vi "Autonomous Independent.vi"() -> ()   [LabVIEW 2015]
doc: "This VI is called when autonomous begins, and will automatically be terminated when autonomous ends. You can carry out timed or sensor driven robot movement independently without needing to return to the caller."
uses:
  Autonomous movements.ctl
  Mode for autonomous.ctl
  <vilib>/Rock Robotics/WPI/Utilities/WPI_GetSetVariantRefNum.vi
  <vilib>/Rock Robotics/Network Tables/NT Read String.vi
  <vilib>/Rock Robotics/Network Tables/NT Write Numeric Array.vi
  <vilib>/Rock Robotics/Network Tables/SD Write String.vi
  <vilib>/Rock Robotics/WPI/RobotDrive/WPI_RobotDriveArcadeDrive_Standard(NoSaturation).vi
  <vilib>/Rock Robotics/Network Tables/SD Write Numeric Array.vi
panel:
  in  "shoot low goal O5 (any)":T1[](array[typedef])=[{"X Joystick Value"=0.0, "Y Joystick Value"=-0.3673469387755101, "Z Joystick Value"=0.0, "Delay (sec)"=4.0, "Movement Name"="", "Mode"=enum."Move Robot"}, {"X Joystick Value"=-0.313131, "Y Joystick Value"=0.0, "Z Joystick Value"=0.0, "Delay (sec)"=1.5, "Movement Name"="", "Mode"=enum."Move Robot"}, {"X Joystick Value"=0.0, "Y Joystick Value"=-0.3, "Z Joystick Value"=0.0, "Delay (sec)"=3.5, "Movement Name"="", "Mode"=enum."Move Robot"}, {"X Joystick Value"=0.373737, "Y Joystick Value"=0.0, "Z Joystick Value"=0.0, "Delay (sec)"=1.5, "Movement Name"="", "Mode"=enum."Move Robot"}, {"X Joystick Value"=0.0, "Y Joystick Value"=-0.3673469387755101, "Z Joystick Value"=0.0, "Delay (sec)"=1.5, "Movement Name"="", "Mode"=enum."Move Robot"}, {"X Joystick Value"=0.0, "Y Joystick Value"=0.0, "Z Joystick Value"=0.0, "Delay (sec)"=2.5, "Movement Name"="", "Mode"=enum."Shoot Low Goal"}, {"X Joystick Value"=0.0, "Y Joystick Value"=-1.0, "Z Joystick Value"=0.0, "Delay (sec)"=0.0, "Movement Name"="", "Mode"=enum."Move Robot"}, {"X Joystick Value"=-1.0, "Y Joystick Value"=0.0, "Z Joystick Value"=0.0, "Delay (sec)"=0.0, "Movement Name"="", "Mode"=enum."Do Nothing"}, {"X Joystick Value"=0.0, "Y Joystick Value"=-1.0, "Z Joystick Value"=0.0, "Delay (sec)"=0.0, "Movement Name"="", "Mode"=enum."Do Nothing"}, {"X Joystick Value"=0.0, "Y Joystick Value"=0.0, "Z Joystick Value"=0.0, "Delay (sec)"=5.0, "Movement Name"="", "Mode"=enum."Do Nothing"}, {"X Joystick Value"=0.0, "Y Joystick Value"=-1.0, "Z Joystick Value"=0.0, "Delay (sec)"=0.0, "Movement Name"="", "Mode"=enum."Do Nothing"}, {"X Joystick Value"=0.0, "Y Joystick Value"=0.0, "Z Joystick Value"=0.0, "Delay (sec)"=0.0, "Movement Name"="", "Mode"=enum."Do Nothing"}] {"Z Joystick Value" scale=-1.0..1.0; "Y Joystick Value" scale=1.0..-1.0; "X Joystick Value" scale=-1.0..1.0}
  in  "shoot low goal O4 (any)":T1[](array[typedef])=[{"X Joystick Value"=0.0, "Y Joystick Value"=-0.3673469387755101, "Z Joystick Value"=0.0, "Delay (sec)"=4.0, "Movement Name"="", "Mode"=enum."Move Robot"}, {"X Joystick Value"=-0.313131, "Y Joystick Value"=0.0, "Z Joystick Value"=0.0, "Delay (sec)"=1.5, "Movement Name"="", "Mode"=enum."Move Robot"}, {"X Joystick Value"=0.0, "Y Joystick Value"=-0.3, "Z Joystick Value"=0.0, "Delay (sec)"=3.5, "Movement Name"="", "Mode"=enum."Move Robot"}, {"X Joystick Value"=0.373737, "Y Joystick Value"=0.0, "Z Joystick Value"=0.0, "Delay (sec)"=0.75, "Movement Name"="", "Mode"=enum."Move Robot"}, {"X Joystick Value"=0.0, "Y Joystick Value"=-0.3673469387755101, "Z Joystick Value"=0.0, "Delay (sec)"=1.5, "Movement Name"="", "Mode"=enum."Move Robot"}, {"X Joystick Value"=0.0, "Y Joystick Value"=0.0, "Z Joystick Value"=0.0, "Delay (sec)"=2.5, "Movement Name"="", "Mode"=enum."Shoot Low Goal"}, {"X Joystick Value"=0.0, "Y Joystick Value"=-1.0, "Z Joystick Value"=0.0, "Delay (sec)"=0.0, "Movement Name"="", "Mode"=enum."Move Robot"}, {"X Joystick Value"=-1.0, "Y Joystick Value"=0.0, "Z Joystick Value"=0.0, "Delay (sec)"=0.0, "Movement Name"="", "Mode"=enum."Do Nothing"}, {"X Joystick Value"=0.0, "Y Joystick Value"=-1.0, "Z Joystick Value"=0.0, "Delay (sec)"=0.0, "Movement Name"="", "Mode"=enum."Do Nothing"}, {"X Joystick Value"=0.0, "Y Joystick Value"=0.0, "Z Joystick Value"=0.0, "Delay (sec)"=5.0, "Movement Name"="", "Mode"=enum."Do Nothing"}, {"X Joystick Value"=0.0, "Y Joystick Value"=-1.0, "Z Joystick Value"=0.0, "Delay (sec)"=0.0, "Movement Name"="", "Mode"=enum."Do Nothing"}, {"X Joystick Value"=0.0, "Y Joystick Value"=0.0, "Z Joystick Value"=0.0, "Delay (sec)"=0.0, "Movement Name"="", "Mode"=enum."Do Nothing"}] {"Z Joystick Value" scale=-1.0..1.0; "Y Joystick Value" scale=1.0..-1.0; "X Joystick Value" scale=-1.0..1.0}
  in  "shoot low goal O3 (any)":T1[](array[typedef])=[{"X Joystick Value"=0.0, "Y Joystick Value"=-0.3673469387755101, "Z Joystick Value"=0.0, "Delay (sec)"=4.0, "Movement Name"="", "Mode"=enum."Move Robot"}, {"X Joystick Value"=0.31313131313131326, "Y Joystick Value"=0.0, "Z Joystick Value"=0.0, "Delay (sec)"=1.5, "Movement Name"="", "Mode"=enum."Move Robot"}, {"X Joystick Value"=0.0, "Y Joystick Value"=-0.3, "Z Joystick Value"=0.0, "Delay (sec)"=3.5, "Movement Name"="", "Mode"=enum."Move Robot"}, {"X Joystick Value"=-0.373737, "Y Joystick Value"=0.0, "Z Joystick Value"=0.0, "Delay (sec)"=0.75, "Movement Name"="", "Mode"=enum."Move Robot"}, {"X Joystick Value"=0.0, "Y Joystick Value"=-0.3673469387755101, "Z Joystick Value"=0.0, "Delay (sec)"=1.5, "Movement Name"="", "Mode"=enum."Move Robot"}, {"X Joystick Value"=0.0, "Y Joystick Value"=0.0, "Z Joystick Value"=0.0, "Delay (sec)"=2.5, "Movement Name"="", "Mode"=enum."Shoot Low Goal"}, {"X Joystick Value"=0.0, "Y Joystick Value"=-1.0, "Z Joystick Value"=0.0, "Delay (sec)"=0.0, "Movement Name"="", "Mode"=enum."Move Robot"}, {"X Joystick Value"=-1.0, "Y Joystick Value"=0.0, "Z Joystick Value"=0.0, "Delay (sec)"=0.0, "Movement Name"="", "Mode"=enum."Do Nothing"}, {"X Joystick Value"=0.0, "Y Joystick Value"=-1.0, "Z Joystick Value"=0.0, "Delay (sec)"=0.0, "Movement Name"="", "Mode"=enum."Do Nothing"}, {"X Joystick Value"=0.0, "Y Joystick Value"=0.0, "Z Joystick Value"=0.0, "Delay (sec)"=5.0, "Movement Name"="", "Mode"=enum."Do Nothing"}, {"X Joystick Value"=0.0, "Y Joystick Value"=-1.0, "Z Joystick Value"=0.0, "Delay (sec)"=0.0, "Movement Name"="", "Mode"=enum."Do Nothing"}, {"X Joystick Value"=0.0, "Y Joystick Value"=0.0, "Z Joystick Value"=0.0, "Delay (sec)"=0.0, "Movement Name"="", "Mode"=enum."Do Nothing"}] {"Z Joystick Value" scale=-1.0..1.0; "Y Joystick Value" scale=1.0..-1.0; "X Joystick Value" scale=-1.0..1.0}
  in  "shoot low goal O2 (any)":T1[](array[typedef])=[{"X Joystick Value"=0.0, "Y Joystick Value"=-0.3673469387755101, "Z Joystick Value"=0.0, "Delay (sec)"=4.0, "Movement Name"="", "Mode"=enum."Move Robot"}, {"X Joystick Value"=0.31313131313131326, "Y Joystick Value"=0.0, "Z Joystick Value"=0.0, "Delay (sec)"=1.5, "Movement Name"="", "Mode"=enum."Move Robot"}, {"X Joystick Value"=0.0, "Y Joystick Value"=-0.3, "Z Joystick Value"=0.0, "Delay (sec)"=3.5, "Movement Name"="", "Mode"=enum."Move Robot"}, {"X Joystick Value"=-0.373737, "Y Joystick Value"=0.0, "Z Joystick Value"=0.0, "Delay (sec)"=1.5, "Movement Name"="", "Mode"=enum."Move Robot"}, {"X Joystick Value"=0.0, "Y Joystick Value"=-0.3673469387755101, "Z Joystick Value"=0.0, "Delay (sec)"=1.5, "Movement Name"="", "Mode"=enum."Move Robot"}, {"X Joystick Value"=0.0, "Y Joystick Value"=0.0, "Z Joystick Value"=0.0, "Delay (sec)"=2.5, "Movement Name"="", "Mode"=enum."Shoot Low Goal"}, {"X Joystick Value"=0.0, "Y Joystick Value"=-1.0, "Z Joystick Value"=0.0, "Delay (sec)"=0.0, "Movement Name"="", "Mode"=enum."Move Robot"}, {"X Joystick Value"=-1.0, "Y Joystick Value"=0.0, "Z Joystick Value"=0.0, "Delay (sec)"=0.0, "Movement Name"="", "Mode"=enum."Do Nothing"}, {"X Joystick Value"=0.0, "Y Joystick Value"=-1.0, "Z Joystick Value"=0.0, "Delay (sec)"=0.0, "Movement Name"="", "Mode"=enum."Do Nothing"}, {"X Joystick Value"=0.0, "Y Joystick Value"=0.0, "Z Joystick Value"=0.0, "Delay (sec)"=5.0, "Movement Name"="", "Mode"=enum."Do Nothing"}, {"X Joystick Value"=0.0, "Y Joystick Value"=-1.0, "Z Joystick Value"=0.0, "Delay (sec)"=0.0, "Movement Name"="", "Mode"=enum."Do Nothing"}, {"X Joystick Value"=0.0, "Y Joystick Value"=0.0, "Z Joystick Value"=0.0, "Delay (sec)"=0.0, "Movement Name"="", "Mode"=enum."Do Nothing"}] {"Z Joystick Value" scale=-1.0..1.0; "Y Joystick Value" scale=1.0..-1.0; "X Joystick Value" scale=-1.0..1.0}
  in  "shoot low goal O1.":T1[](array[typedef])=[{"X Joystick Value"=0.0, "Y Joystick Value"=-0.3673469387755101, "Z Joystick Value"=0.0, "Delay (sec)"=4.0, "Movement Name"="", "Mode"=enum."Move Robot"}, {"X Joystick Value"=0.31313131313131326, "Y Joystick Value"=0.0, "Z Joystick Value"=0.0, "Delay (sec)"=1.5, "Movement Name"="", "Mode"=enum."Move Robot"}, {"X Joystick Value"=0.0, "Y Joystick Value"=-0.3, "Z Joystick Value"=0.0, "Delay (sec)"=4.0, "Movement Name"="", "Mode"=enum."Move Robot"}, {"X Joystick Value"=-0.373737, "Y Joystick Value"=0.0, "Z Joystick Value"=0.0, "Delay (sec)"=1.5, "Movement Name"="", "Mode"=enum."Move Robot"}, {"X Joystick Value"=0.0, "Y Joystick Value"=-0.3673469387755101, "Z Joystick Value"=0.0, "Delay (sec)"=1.5, "Movement Name"="", "Mode"=enum."Move Robot"}, {"X Joystick Value"=0.0, "Y Joystick Value"=0.0, "Z Joystick Value"=0.0, "Delay (sec)"=2.5, "Movement Name"="", "Mode"=enum."Shoot Low Goal"}, {"X Joystick Value"=0.0, "Y Joystick Value"=-1.0, "Z Joystick Value"=0.0, "Delay (sec)"=0.0, "Movement Name"="", "Mode"=enum."Move Robot"}, {"X Joystick Value"=-1.0, "Y Joystick Value"=0.0, "Z Joystick Value"=0.0, "Delay (sec)"=0.0, "Movement Name"="", "Mode"=enum."Do Nothing"}, {"X Joystick Value"=0.0, "Y Joystick Value"=-1.0, "Z Joystick Value"=0.0, "Delay (sec)"=0.0, "Movement Name"="", "Mode"=enum."Do Nothing"}, {"X Joystick Value"=0.0, "Y Joystick Value"=0.0, "Z Joystick Value"=0.0, "Delay (sec)"=5.0, "Movement Name"="", "Mode"=enum."Do Nothing"}, {"X Joystick Value"=0.0, "Y Joystick Value"=-1.0, "Z Joystick Value"=0.0, "Delay (sec)"=0.0, "Movement Name"="", "Mode"=enum."Do Nothing"}, {"X Joystick Value"=0.0, "Y Joystick Value"=0.0, "Z Joystick Value"=0.0, "Delay (sec)"=0.0, "Movement Name"="", "Mode"=enum."Do Nothing"}] {"Z Joystick Value" scale=-1.0..1.0; "Y Joystick Value" scale=1.0..-1.0; "X Joystick Value" scale=-1.0..1.0}
  in  "move forward":T1[](array[typedef])=[{"X Joystick Value"=0.0, "Y Joystick Value"=-0.3, "Z Joystick Value"=0.0, "Delay (sec)"=2.5, "Movement Name"="", "Mode"=enum."Move Robot"}, {"X Joystick Value"=0.0, "Y Joystick Value"=0.0, "Z Joystick Value"=0.0, "Delay (sec)"=5.0, "Movement Name"="", "Mode"=enum."Move Robot"}, {"X Joystick Value"=0.0, "Y Joystick Value"=-1.0, "Z Joystick Value"=0.0, "Delay (sec)"=0.0, "Movement Name"="", "Mode"=enum."Move Robot"}, {"X Joystick Value"=-1.0, "Y Joystick Value"=0.0, "Z Joystick Value"=0.0, "Delay (sec)"=5.0, "Movement Name"="", "Mode"=enum."Do Nothing"}, {"X Joystick Value"=0.0, "Y Joystick Value"=-1.0, "Z Joystick Value"=0.0, "Delay (sec)"=0.0, "Movement Name"="", "Mode"=enum."Do Nothing"}, {"X Joystick Value"=0.0, "Y Joystick Value"=0.0, "Z Joystick Value"=0.0, "Delay (sec)"=0.0, "Movement Name"="", "Mode"=enum."Do Nothing"}, {"X Joystick Value"=0.0, "Y Joystick Value"=-1.0, "Z Joystick Value"=0.0, "Delay (sec)"=0.0, "Movement Name"="", "Mode"=enum."Move Robot"}, {"X Joystick Value"=-1.0, "Y Joystick Value"=0.0, "Z Joystick Value"=0.0, "Delay (sec)"=0.0, "Movement Name"="", "Mode"=enum."Do Nothing"}, {"X Joystick Value"=0.0, "Y Joystick Value"=-1.0, "Z Joystick Value"=0.0, "Delay (sec)"=0.0, "Movement Name"="", "Mode"=enum."Do Nothing"}, {"X Joystick Value"=0.0, "Y Joystick Value"=0.0, "Z Joystick Value"=0.0, "Delay (sec)"=5.0, "Movement Name"="", "Mode"=enum."Do Nothing"}, {"X Joystick Value"=0.0, "Y Joystick Value"=-1.0, "Z Joystick Value"=0.0, "Delay (sec)"=0.0, "Movement Name"="", "Mode"=enum."Do Nothing"}, {"X Joystick Value"=0.0, "Y Joystick Value"=0.0, "Z Joystick Value"=0.0, "Delay (sec)"=0.0, "Movement Name"="", "Mode"=enum."Do Nothing"}] {"Z Joystick Value" scale=-1.0..1.0; "Y Joystick Value" scale=1.0..-1.0; "X Joystick Value" scale=-1.0..1.0}
  in  "do nothing":T1[](array[typedef])=[{"X Joystick Value"=0.0, "Y Joystick Value"=0.0, "Z Joystick Value"=0.0, "Delay (sec)"=15.0, "Movement Name"="", "Mode"=enum."Do Nothing"}] {"Z Joystick Value" scale=-1.0..1.0; "Y Joystick Value" scale=1.0..-1.0; "X Joystick Value" scale=-1.0..1.0}
  out "Current Movement, for debugging":T3 {"Y Joystick Value" scale=1.0..-1.0; "X Joystick Value" scale=-1.0..1.0}
  in  "Array of robot movements":T4(array[cluster])=[{"X Joystick Value"=0.39393939393939403, "Y Joystick Value"=0.0, "Delay (sec)"=1.0, "Movement Name"="turn"}, {"X Joystick Value"=-0.3737373737373737, "Y Joystick Value"=0.0, "Delay (sec)"=1.0, "Movement Name"="turn back"}] {"Y Joystick Value" scale=1.0..-1.0; "X Joystick Value" scale=-1.0..1.0}
  # "Be sure to right-click and choose Data Operations>>Make Current Value default if you want to save the array values with the VI"
  # "start in position one"
  # "DONT USE Z VALUE\n\nSET CURRENT VALUES AS DEFAULT"
  # "move forward"
  # "shoot low goal"
  # "move forward"
  # "turn left"
  # "turn right"
  # "move forward"
  # "move forward"
  # "turn right"
  # "move forward"
  # "turn left"
  # "shoot low goal"
  # "move forward"
  # "move forward"
  # "turn right"
  # "move forward"
  # "turn left"
  # "shoot low goal"
  # "move forward"
  # "move forward"
  # "turn left"
  # "move forward"
  # "turn right"
  # "shoot low goal"
  # "move forward"
  # "move forward"
  # "move forward"
  # "turn left"
  # "move forward"
  # "turn right"
  # "shoot low goal"
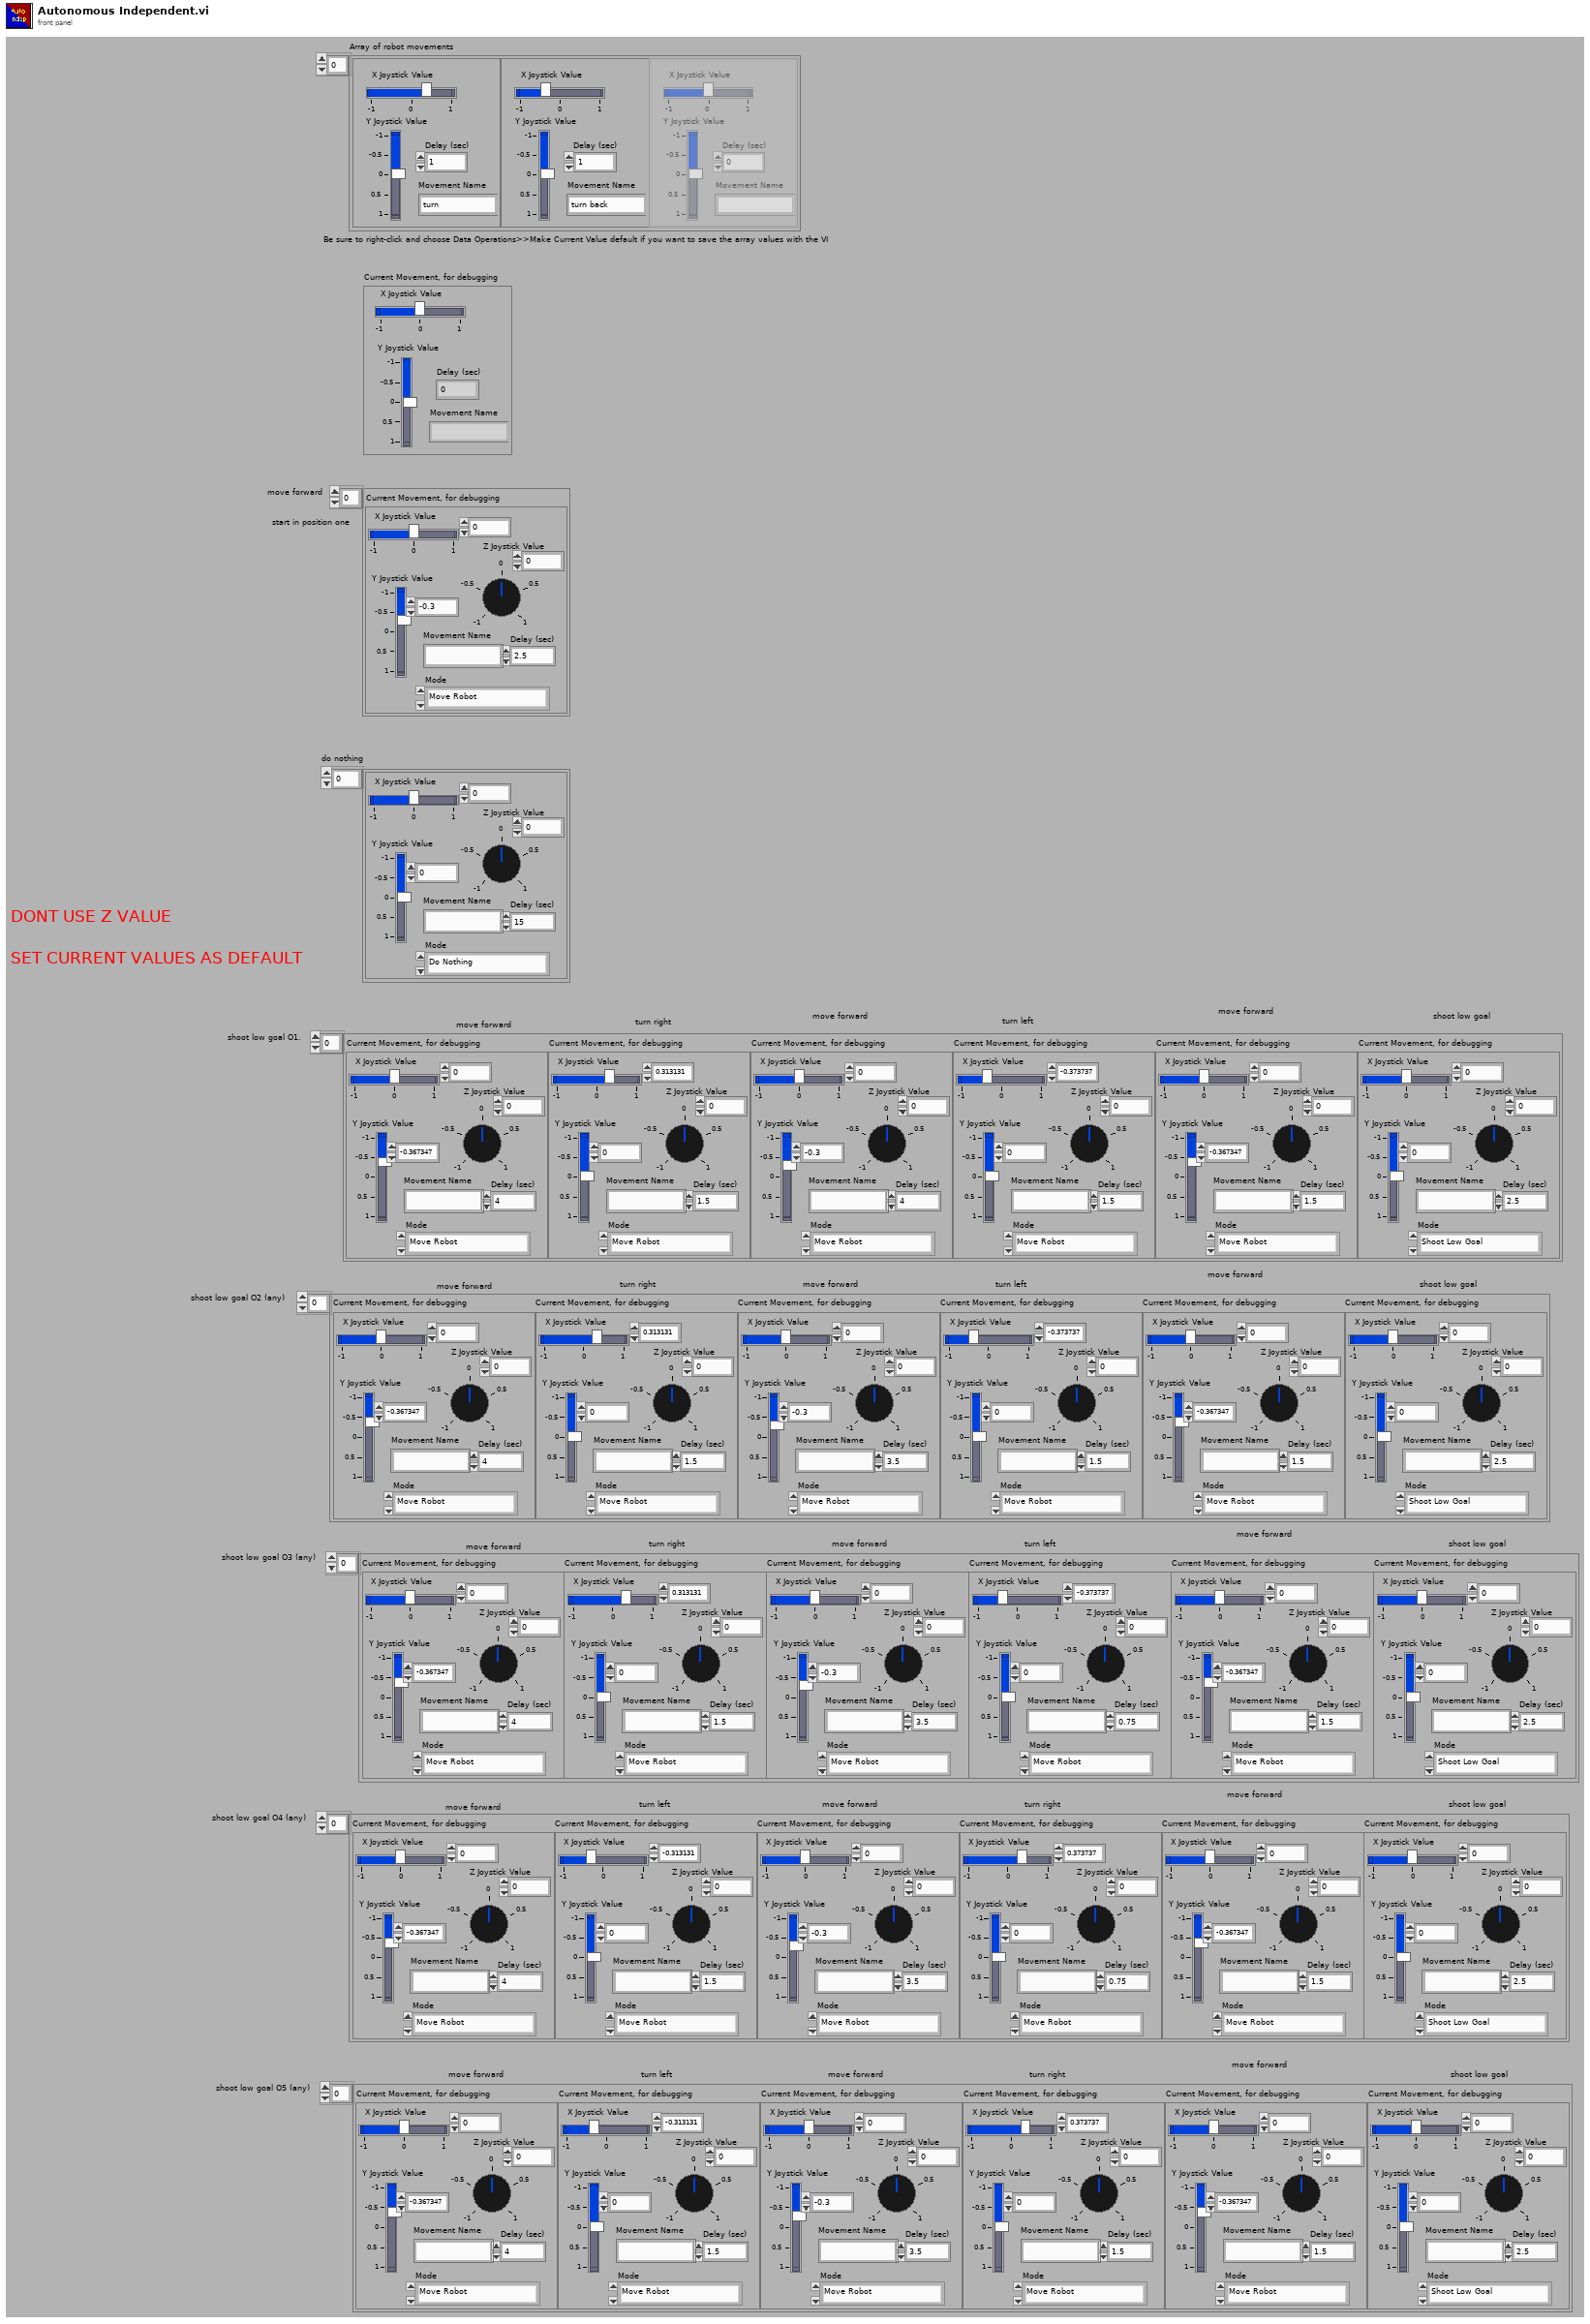
[diagram p1: front panel]
types:
  T1 = typedef "Autonomous movements.ctl" = cluster{"X Joystick Value":dbl, "Y Joystick Value":dbl, "Z Joystick Value":dbl, "Delay (sec)":dbl, "Movement Name":string, "Mode":T2}
  T2 = typedef "Mode for autonomous.ctl" = enum16{"Do Nothing", "Move Robot", "Shoot Low Goal", "Shoot High Goal"}
  T3 = cluster{"X Joystick Value":dbl, "Y Joystick Value":dbl, "Delay (sec)":dbl, "Movement Name":string}
  T4 = cluster{"X Joystick Value":dbl, "Y Joystick Value":dbl, "Delay (sec)":dbl, "Movement Name":string}[]
  T5 = typedef "WPI_JoystickDevRef.ctl" = cluster{"Device":T6}
  T6 = typedef "WPI_JoystickDeviceEnum.ctl" = enum16{"USB 0", "USB 1", "USB 2", "USB 3", "USB 4", "USB 5"}
  T7 = typedef "WPI_RobotDriveDevRef.ctl" = cluster{"DevStatus":errorcluster, "Motors[]":T8[], "Square Inputs":bool, "Max Output":dbl}
  T8 = typedef "WPI_MotorControlDeviceRef.ctl" = cluster{"DeviceStatus":errorcluster, "Type":T9, "PWM":cluster{"PWM Channel":T10, "DeadBand":T11}, "CAN":cluster{"Device Number":u8, "Control Mode":T12, "Semaphore":T13, "Max Vout":dbl, "TalonSRX Control Mode":T14}, "Invert":bool}
  T9 = typedef "WPI_MotorControlType.ctl" = enum16{"PWM", "CAN", "CANTalonSRX"}
  T10 = typedef "FPGA_DIOPWMChannel.ctl" = enum8{"PWM 0", "PWM 1", "PWM 2", "PWM 3", "PWM 4", "PWM 5", "PWM 6", "PWM 7", "PWM 8", "PWM 9", "PWM MXP 0", "PWM MXP 1", "PWM MXP 2", "PWM MXP 3", "PWM MXP 4", "PWM MXP 5", "PWM MXP 6", "PWM MXP 7", "PWM MXP 8", "PWM MXP 9", "Invalid"}
  T11 = typedef "WPI_PWMDeadband.ctl" = cluster{"Name":string, "maxPositivePwm":i32, "minPositivePwm":i32, "centerPwm":i32, "maxNegativePwm":i32, "minNegativePwm":i32, "angularRange":u16}
  T12 = typedef "WPI_CANJaguar_ControlMode.ctl" = enum8{"Percent VBus", "Current", "Speed", "Position", "Voltage"}
  T13 = typedef "Semaphore RefNum" = refnum<k1>
  T14 = typedef "WPI_CANTalonSRX_APIControlMode.ctl" = enum8{"Percent VBus", "Speed", "Position", "Slave", "Unchanged / Invalid", "Voltage Compensation", "Current", "Motion Profile"}
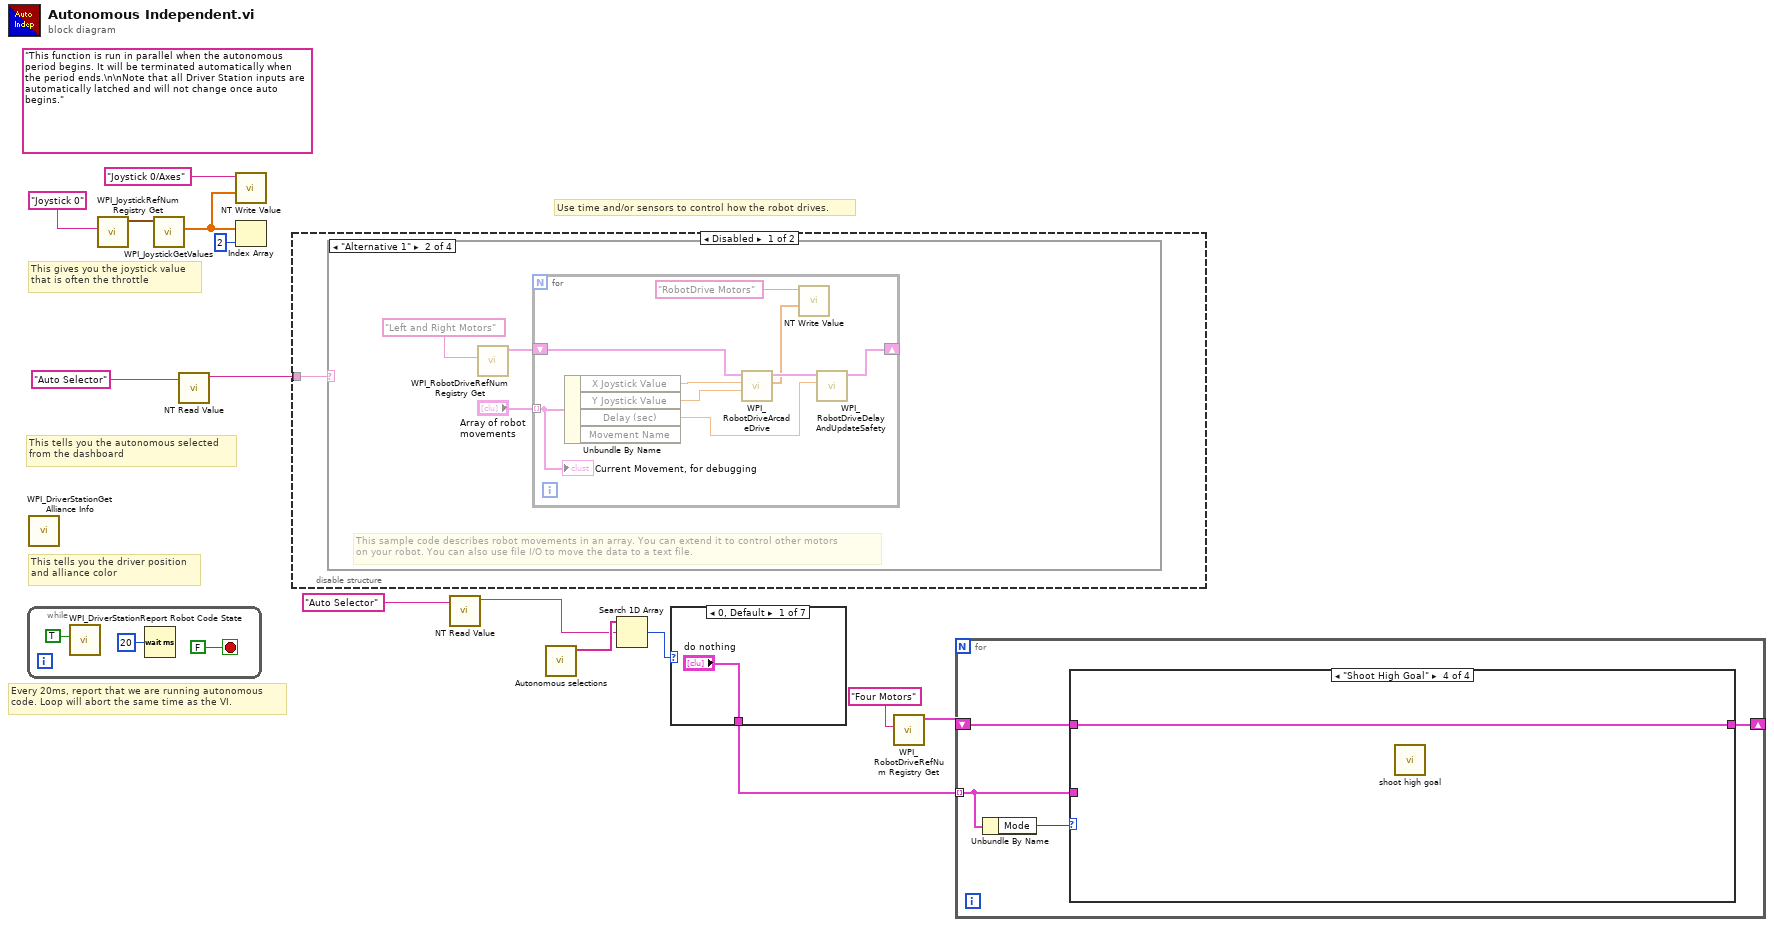
[diagram p0: block diagram]
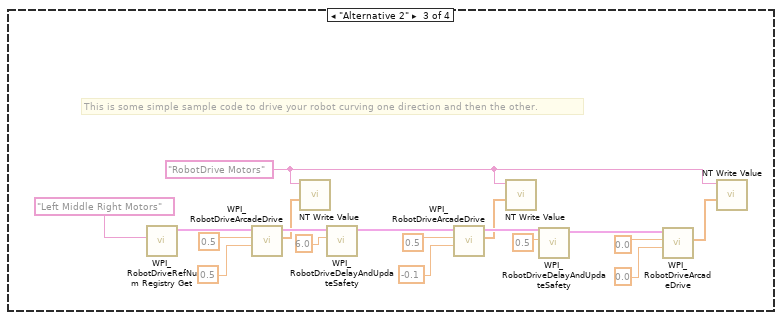
[diagram p3: hidden frame]
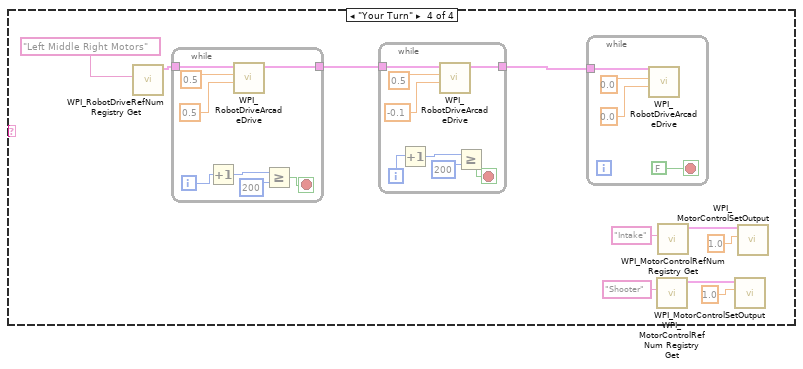
[diagram p4: hidden frame]
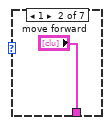
[diagram p6: hidden frame]
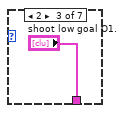
[diagram p7: hidden frame]
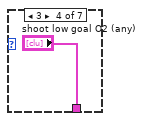
[diagram p8: hidden frame]
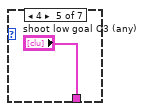
[diagram p9: hidden frame]
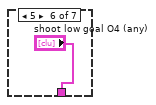
[diagram p10: hidden frame]
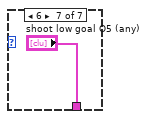
[diagram p11: hidden frame]
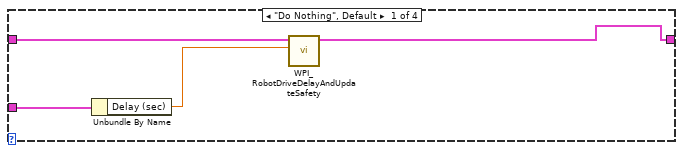
[diagram p12: hidden frame]
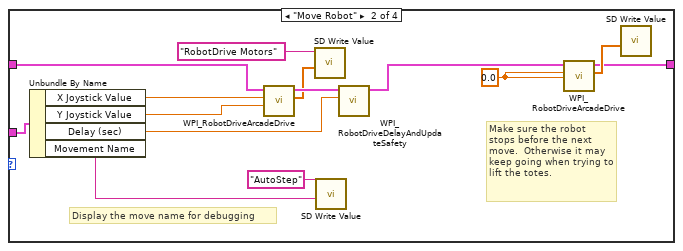
[diagram p13: hidden frame]
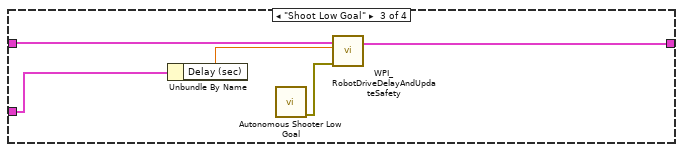
[diagram p14: hidden frame]
diagram:
  (unwired) "This function is run in parallel when the autonomous period begins. It will be terminated automatically when the period ends.\n\nNote that all Driver Station inputs are automatically latched and will not change once auto begins."
  # "This tells you the autonomous selected\nfrom the dashboard"
  # "Every 20ms, report that we are running autonomous\ncode. Loop will abort the same time as the VI."
  # "This gives you the joystick value\nthat is often the throttle"
  # "Use time and/or sensors to control how the robot drives."
  # "This tells you the driver position\nand alliance color"
  n1 = while {
    stop <- FALSE stop-if-true
    n2 = call <vilib>:"WPI_DriverStationReport Robot Code State.vi"("Autonomous"=TRUE) -> ()  [unwired: 10 in, 1 out]
    n3 = Wait (ms)(milliseconds to wait=u32 20) -> ()  [unwired: 1 out]
  }
  n4 = call <vilib>:"WPI_DriverStationGet Alliance Info.vi"() -> ()  [unwired: 12 out]
  n5 = call <vilib>:"WPI_JoystickRefNum Registry Get.vi"("refnum name"="Joystick 0") -> ("JoystickDevRef"=w13:T5)  [unwired: 1 in, 9 out]
  n6 = call <vilib>:"WPI_JoystickGetValues.vi"("JoystickDevRef"=w13) -> ("Axes"=w9:dbl[])  [unwired: 6 in, 4 out]
  n7 = call-poly <vilib>:"NT Read Value.vi"("Name"="Auto Selector") -> ("String"=w10:string)  [unwired: 9 in, 1 out]
  n8 = call-poly <vilib>:"NT Write Value.vi"("Numeric Array"=w9, "Name"="Joystick 0/Axes") -> ()  [unwired: 9 in, 1 out]
  n9 = Index Array(array=w9, index=2) -> ()  [unwired: 1 out]
  n10 = disable-structure shown="Disabled" {
    disable-tunnel: w10 -> [w18 _]
    frame Disabled {
      n11 = case shown="\"Alternative 1\"" w18 {
        frame Default {
          # "You can put your main auto here, or you can right-click on the case and make any\nother frame be the default case."
          # "This is the frame that will execute if no selection is made, or if it is not recognized"
        }
        frame "Alternative 1" {
          # "This sample code describes robot movements in an array. You can extend it to control other motors\non your robot. You can also use file I/O to move the data to a text file."
          n12 = call <vilib>:"WPI_RobotDriveRefNum Registry Get.vi"("refnum name"="Left and Right Motors") -> ("RobotDriveDevRef"=w20:T7)  [unwired: 1 in, 9 out]
          n13 = for {
            shift-right: [w28] -> _
            shift-left: w20 -> [w29]
            tunnel: "Array of robot movements" -> [w24] mode=indexing
            n14 = Unbundle By Name(w24) -> ("X Joystick Value"=w27:dbl, "Y Joystick Value"=w26:dbl, "Delay (sec)"=w25:dbl)  [unwired: 1 out]
            n15 = call-poly <vilib>:"WPI_RobotDriveArcadeDrive.vi"("Y axis value"=w26, "X axis value"=w27, "RobotDriveDevRef"=w29) -> ("Motor Values"=w22:dbl[], "RobotDriveDevRef"=w30:T7)  [unwired: 1 in, 6 out]
            n16 = call-poly <vilib>:"NT Write Value.vi"("Numeric Array"=w22, "Name"="RobotDrive Motors") -> ()  [unwired: 9 in, 1 out]
            n17 = call <vilib>:"WPI_RobotDriveDelayAndUpdateSafety.vi"("Delay (s)"=w25, "RobotDriveDevRef"=w30) -> ("RobotDriveDevRef 2"=w28:T7)  [unwired: 8 in, 1 out]
            "Current Movement, for debugging" <- w24
          }
        }
        frame "Alternative 2" {
          w32 = "RobotDrive Motors" ("Name")
          # "This is some simple sample code to drive your robot curving one direction and then the other."
          n18 = call <vilib>:"WPI_RobotDriveRefNum Registry Get.vi"("refnum name"="Left Middle Right Motors") -> ("RobotDriveDevRef"=w48:T7)  [unwired: 1 in, 9 out]
          n19 = call-poly <vilib>:"WPI_RobotDriveArcadeDrive.vi"("Y axis value"=0.5 ("X axis value"), "X axis value"=0.5, "RobotDriveDevRef"=w48) -> ("Motor Values"=w31:dbl[], "RobotDriveDevRef"=w41:T7)  [unwired: 1 in, 6 out]
          n20 = call-poly <vilib>:"NT Write Value.vi"("Numeric Array"=w31, "Name"=w32) -> ()  [unwired: 9 in, 1 out]
          n21 = call <vilib>:"WPI_RobotDriveDelayAndUpdateSafety.vi"("Delay (s)"=6.0, "RobotDriveDevRef"=w41) -> ("RobotDriveDevRef 2"=w42:T7)  [unwired: 8 in, 1 out]
          n22 = call-poly <vilib>:"WPI_RobotDriveArcadeDrive.vi"("Y axis value"=-0.1 ("X axis value"), "X axis value"=0.5, "RobotDriveDevRef"=w42) -> ("Motor Values"=w33:dbl[], "RobotDriveDevRef"=w43:T7)  [unwired: 1 in, 6 out]
          n23 = call-poly <vilib>:"NT Write Value.vi"("Numeric Array"=w33, "Name"=w32) -> ()  [unwired: 9 in, 1 out]
          n24 = call <vilib>:"WPI_RobotDriveDelayAndUpdateSafety.vi"("Delay (s)"=0.5, "RobotDriveDevRef"=w43) -> ("RobotDriveDevRef 2"=w44:T7)  [unwired: 8 in, 1 out]
          n25 = call-poly <vilib>:"WPI_RobotDriveArcadeDrive.vi"("Y axis value"=0.0 ("X axis value"), "X axis value"=0.0, "RobotDriveDevRef"=w44) -> ("Motor Values"=w34:dbl[])  [unwired: 1 in, 7 out]
          n26 = call-poly <vilib>:"NT Write Value.vi"("Numeric Array"=w34, "Name"=w32) -> ()  [unwired: 9 in, 1 out]
        }
        frame "Your Turn" {
          n27 = call <vilib>:"WPI_RobotDriveRefNum Registry Get.vi"("refnum name"="Left Middle Right Motors") -> ("RobotDriveDevRef"=w58:T7)  [unwired: 1 in, 9 out]
          n28 = while {
            tunnel: w58 -> [w78]
            tunnel: [w75] -> w50
            i -> [w74]
            stop <- w71 stop-if-true
            n29 = Increment(x=w74) -> (x+1=w73:i32)
            n30 = call-poly <vilib>:"WPI_RobotDriveArcadeDrive.vi"("Y axis value"=0.5 ("X axis value"), "X axis value"=0.5, "RobotDriveDevRef"=w78) -> ("RobotDriveDevRef"=w75:T7)  [unwired: 1 in, 7 out]
            n31 = Greater Or Equal?(x=w73, y=200) -> (x >= y?=w71:bool)
          }
          n32 = while {
            tunnel: w50 -> [w68]
            tunnel: [w67] -> w49
            i -> [w64]
            stop <- w63 stop-if-true
            n33 = Increment(x=w64) -> (x+1=w66:i32)
            n34 = call-poly <vilib>:"WPI_RobotDriveArcadeDrive.vi"("Y axis value"=-0.1 ("X axis value"), "X axis value"=0.5, "RobotDriveDevRef"=w68) -> ("RobotDriveDevRef"=w67:T7)  [unwired: 1 in, 7 out]
            n35 = Greater Or Equal?(x=w66, y=200) -> (x >= y?=w63:bool)
          }
          n36 = while {
            tunnel: w49 -> [w60]
            stop <- FALSE stop-if-true
            n37 = call-poly <vilib>:"WPI_RobotDriveArcadeDrive.vi"("Y axis value"=0.0 ("X axis value"), "X axis value"=0.0, "RobotDriveDevRef"=w60) -> ()  [unwired: 1 in, 8 out]
          }
          n38 = call <vilib>:"WPI_MotorControlRefNum Registry Get.vi"("refnum name"="Shooter") -> ("MotorControlDevRef"=w55:T8)  [unwired: 9 in, 1 out]
          n39 = call <vilib>:"WPI_MotorControlRefNum Registry Get.vi"("refnum name"="Intake") -> ("MotorControlDevRef"=w52:T8)  [unwired: 9 in, 1 out]
          n40 = call <vilib>:"WPI_MotorControlSetOutput.vi"("Output"=1.0, "MotorControlDevRef"=w55) -> ()  [unwired: 7 in, 3 out]
          n41 = call <vilib>:"WPI_MotorControlSetOutput.vi"("Output"=1.0, "MotorControlDevRef"=w52) -> ()  [unwired: 7 in, 3 out]
        }
      }
    }
    frame Enabled {
    }
  }
  n42 = call-poly <vilib>:"NT Read Value.vi"("Name"="Auto Selector") -> ("String"=w2:string)  [unwired: 9 in, 1 out]
  n43 = call "Autonomous selections.vi"() -> ("Autonomous selections"=w3:string[])  [unwired: 11 in]
  n44 = Search 1D Array(1D array=w3, element=w2) -> (index of element=w1:i32)  [unwired: 1 in]
  n45 = case shown="0, Default" w1 {
    tunnel: ["do nothing" "move forward" "shoot low goal O1." "shoot low goal O2 (any)" "shoot low goal O3 (any)" "shoot low goal O4 (any)" "shoot low goal O5 (any)"] -> w4
    frame 0, Default {
    }
    frame 1 {
    }
    frame 2 {
    }
    frame 3 {
    }
    frame 4 {
    }
    frame 5 {
    }
    frame 6 {
    }
  }
  n46 = call <vilib>:"WPI_RobotDriveRefNum Registry Get.vi"("refnum name"="Four Motors") -> ("RobotDriveDevRef"=w6:T7)  [unwired: 1 in, 9 out]
  n47 = for {
    shift-right: [w88] -> _
    shift-left: w6 -> [w89]
    tunnel: w4 -> [w87] mode=indexing
    n48 = Unbundle By Name(w87) -> ("Mode"=w86:T2)
    n49 = case shown="\"Shoot High Goal\"" w86 {
      tunnel: w89 -> [w93 w106 w110 w113]
      tunnel: w87 -> [w92 w102 w111 _]
      tunnel: [w90 w94 w109 w113] -> w88
      frame "Do Nothing", Default {
        n50 = Unbundle By Name(w92) -> ("Delay (sec)"=w91:dbl)
        n51 = call <vilib>:"WPI_RobotDriveDelayAndUpdateSafety.vi"("Delay (s)"=w91, "RobotDriveDevRef"=w93) -> ("RobotDriveDevRef 2"=w90:T7)  [unwired: 8 in, 1 out]
      }
      frame "Move Robot" {
        w95 = 0.0 ("X")
        # "Display the move name for debugging"
        # "Make sure the robot stops before the next move.  Otherwise it may keep going when trying to lift the totes."
        n52 = Unbundle By Name(w102) -> ("X Joystick Value"=w105:dbl, "Y Joystick Value"=w104:dbl, "Delay (sec)"=w103:dbl, "Movement Name"=w100:string)
        n53 = call-poly <vilib>:"WPI_RobotDriveArcadeDrive.vi"("Y axis value"=w104, "X axis value"=w105, "RobotDriveDevRef"=w106) -> ("Motor Values"=w101:dbl[], "RobotDriveDevRef"=w107:T7)  [unwired: 6 in, 1 out]
        n54 = call-poly <vilib>:"SD Write Value.vi"("Numeric Array"=w101, "Name"="RobotDrive Motors") -> ()  [unwired: 8 in, 2 out]
        n55 = call-poly <vilib>:"SD Write Value.vi"("String"=w100, "Name"="AutoStep") -> ()  [unwired: 8 in, 2 out]
        n56 = call <vilib>:"WPI_RobotDriveDelayAndUpdateSafety.vi"("Delay (s)"=w103, "RobotDriveDevRef"=w107) -> ("RobotDriveDevRef 2"=w98:T7)  [unwired: 8 in, 1 out]
        n57 = call-poly <vilib>:"WPI_RobotDriveArcadeDrive.vi"("Y axis value"=w95, "X axis value"=w95, "RobotDriveDevRef"=w98) -> ("Motor Values"=w96:dbl[], "RobotDriveDevRef"=w94:T7)  [unwired: 6 in, 1 out]
        n58 = call-poly <vilib>:"SD Write Value.vi"("Numeric Array"=w96) -> ()  [unwired: 9 in, 2 out]
      }
      frame "Shoot Low Goal" {
        n59 = Unbundle By Name(w111) -> ("Delay (sec)"=w112:dbl)
        n60 = call "Autonomous Shooter Low Goal.vi"() -> ("error out"=w108:errorcluster)  [unwired: 11 in]
        n61 = call <vilib>:"WPI_RobotDriveDelayAndUpdateSafety.vi"("error in (no error)"=w108, "Delay (s)"=w112, "RobotDriveDevRef"=w110) -> ("RobotDriveDevRef 2"=w109:T7)  [unwired: 7 in, 1 out]
      }
      frame "Shoot High Goal" {
        n62 = call "shoot high goal.vi"() -> ()  [unwired: 11 in, 1 out]
      }
    }
  }
